vi "Close.vi"(8 "error in (no error)":errorcluster, 11 "Guardian Subpanel in":refnum<class "Guardian Subpanel.lvclass">) -> (0 "error out":errorcluster, 3 "Guardian Subpanel out":refnum<class "Guardian Subpanel.lvclass">)   [LabVIEW 2026, in "TALOS.lvlib" / "Guardian Subpanel.lvlib" / "Guardian Subpanel.lvclass"]
uses:
  Guardian Subpanel.lvclass
  Father of all uServices/Father of all uServices/Father of all uServices.lvclass
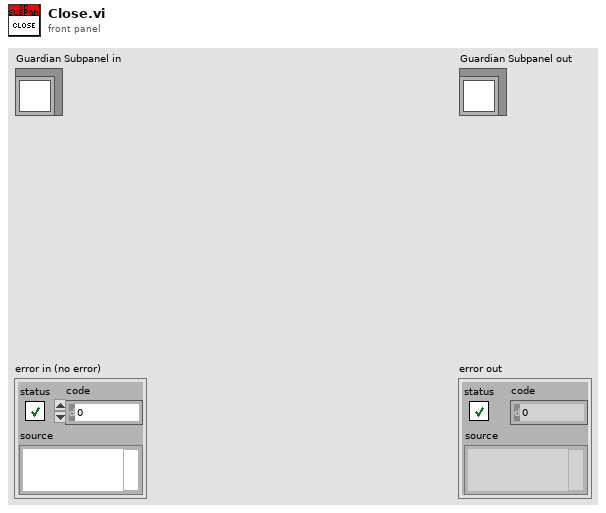
[diagram p1: front panel]
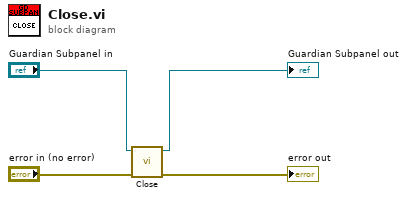
[diagram p0: block diagram]
diagram:
  n1 = call-parent "Close.vi"("error in (no error)"="error in (no error)", "uService Template in"="Guardian Subpanel in") -> ("error out"=→"error out":errorcluster, "uService Template out"=→"Guardian Subpanel out":refnum<class "Guardian Subpanel.lvclass">)  [unwired: 8 in]
